vi "Gamepad Button Map.vi"(1 "Joystick Name":string="Right Joystick") -> (0 "Actions":T1)   [LabVIEW 2012]
uses:
  <vilib>/Rock Robotics/WPI/Joystick/WPI_JoystickGetSetRefNum.vi
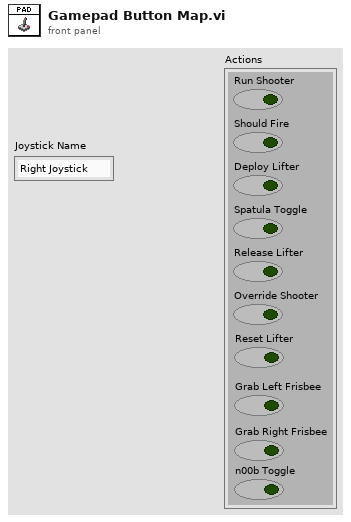
[diagram p1: front panel]
types:
  T1 = cluster{"Run Shooter":bool, "Should Fire":bool, "Deploy Lifter":bool, "Spatula Toggle":bool, "Release Lifter":bool, "Override Shooter":bool, "Reset Lifter":bool, "Grab Left Frisbee":bool, "Grab Right Frisbee":bool, "n00b Toggle":bool}
  T2 = typedef "WPI_JoystickDevRef.ctl" = cluster{"Device":T3}
  T3 = typedef "WPI_JoystickDeviceEnum.ctl" = enum16{"USB 1", "USB 2", "USB 3", "USB 4", "Kinect 1", "Kinect 2"}
  T4 = typedef "WPI_JoystickButtonState.ctl" = cluster{"Button 1":bool, "Button 2":bool, "Button 3":bool, "Button 4":bool, "Button 5":bool, "Button 6":bool, "Button 7":bool, "Button 8":bool, "Button 9":bool, "Button 10":bool, "Button 11":bool, "Button 12":bool}
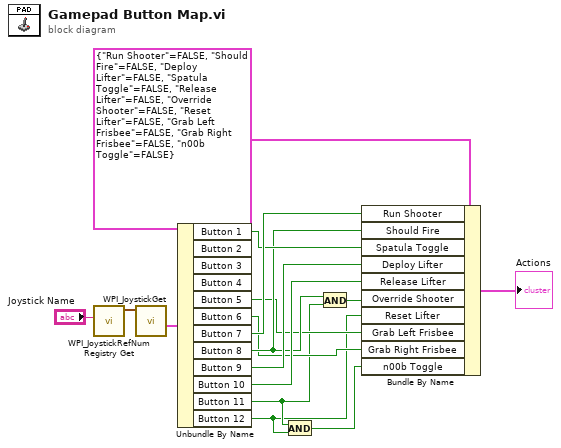
[diagram p0: block diagram]
diagram:
  n1 = call <vilib>:"WPI_JoystickRefNum Registry Get.vi"("refnum name"="Joystick Name") -> ("JoystickDevRef"=w16:T2)  [unwired: 1 in, 9 out]
  n2 = call <vilib>:"WPI_JoystickGet.vi"("JoystickDevRef"=w16) -> ("Buttons"=w14:T4)  [unwired: 1 in, 5 out]
  n3 = Unbundle By Name(w14) -> ("Button 1"=w11:bool, "Button 5"=w6:bool, "Button 6"=w5:bool, "Button 7"=w12:bool, "Button 8"=w7:bool, "Button 9"=w10:bool, "Button 10"=w9:bool, "Button 11"=w3:bool, "Button 12"=w2:bool)  [unwired: 3 out]
  n4 = And(x=w3, y=w2) -> (x .and. y?=w1:bool)
  n5 = And(x=w7, y=w3) -> (x .and. y?=w8:bool)
  n6 = Bundle By Name(cluster=T1 {"Run Shooter"=FALSE, "Should Fire"=FALSE, "Deploy Lifter"=FALSE, "Spatula Toggle"=FALSE, "Release Lifter"=FALSE, "Override Shooter"=FALSE, "Reset Lifter"=FALSE, "Grab Left Frisbee"=FALSE, "Grab Right Frisbee"=FALSE, "n00b Toggle"=FALSE}, "Run Shooter"=w12, "Should Fire"=w7, "Spatula Toggle"=w11, "Deploy Lifter"=w10, "Release Lifter"=w9, "Override Shooter"=w8, "Reset Lifter"=w2, "Grab Left Frisbee"=w6, "Grab Right Frisbee"=w5, "n00b Toggle"=w1) -> (→"Actions":T1)
